vi "StateTurret.vi"(0 "Master State":enum16{"Normal", "Climb"}(ring)) -> ()   [LabVIEW 2020]
doc: "Performs all of the caluclations and decisions related to the turret."
uses:
  sensordata.vi
  robotoutputs.vi
panel:
  in  "Soft Limit A":dbl=125.0
  in  "Soft Limit B":dbl=-139.0
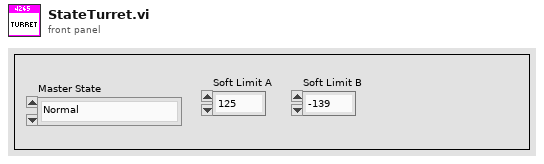
[diagram p1: front panel]
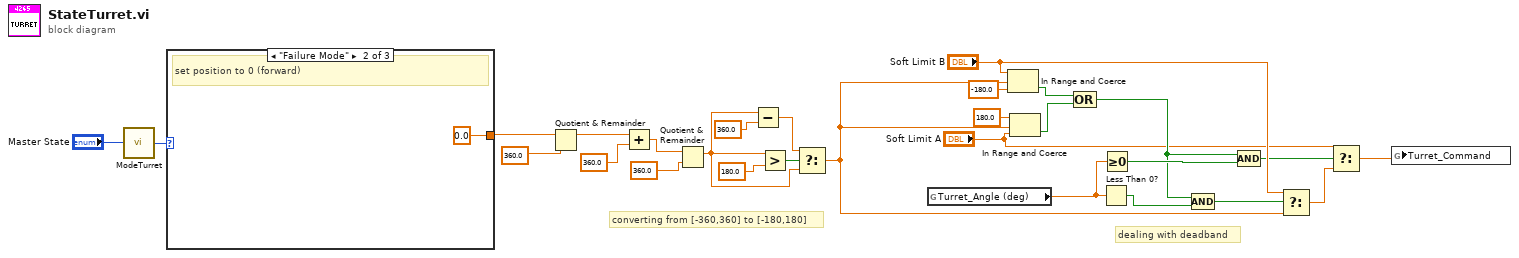
[diagram p0: block diagram]
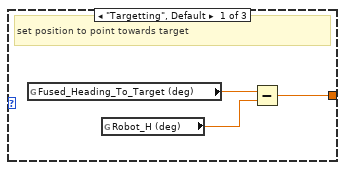
[diagram p2: hidden frame]
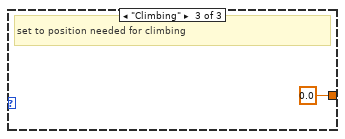
[diagram p3: hidden frame]
diagram:
  # "dealing with deadband"
  # "converting from [-360,360] to [-180,180]"
  n1 = call "ModeTurret.vi"("Master State"="Master State") -> ("Turret Mode"=w28:enum16{"Targetting", "Failure Mode", "Climbing"})
  n2 = case shown="\"Failure Mode\"" w28 {
    tunnel: [w30 0.0 0.0] -> w6
    frame "Targetting", Default {
      # "set position to point towards target"
      n3 = global read "sensordata.vi" "Fused_Heading_To_Target (deg)"() -> (w29:dbl)
      n4 = global read "sensordata.vi" "Robot_H (deg)"() -> (w31:dbl)
      n5 = Subtract(x=w29, y=w31) -> (x-y=w30:dbl)
    }
    frame "Failure Mode" {
      # "set position to 0 (forward)"
    }
    frame "Climbing" {
      # "set to position needed for climbing"
    }
  }
  n6 = Quotient & Remainder(x=w6, y=360.0) -> (x-y*floor(x/y)=w16:dbl)  [unwired: 1 out]
  n7 = Add(x=w16, y=360.0) -> (x+y=w14:dbl)
  n8 = Quotient & Remainder(x=w14, y=360.0) -> (x-y*floor(x/y)=w8:dbl)  [unwired: 1 out]
  n9 = Subtract(x=w8, y=360.0) -> (x-y=w9:dbl)
  n10 = Greater?(x=w8, y=180.0) -> (0:w11:bool)
  n11 = Select(t=w9, s=w11, f=w8) -> (s? t:f=w3:dbl)
  n12 = global read "sensordata.vi" "Turret_Angle (deg)"() -> (w7:dbl)
  n13 = In Range and Coerce(upper limit="Soft Limit B", x=w3, lower limit=-180.0) -> (In Range?=w24:bool)  [unwired: 1 out]
  n14 = In Range and Coerce(upper limit=180.0 ("lower limit"), x=w3, lower limit="Soft Limit A") -> (In Range?=w23:bool)  [unwired: 1 out]
  n15 = Compound Arithmetic op=OR(w24, w23) -> (w22:bool)
  n16 = Less Than 0?(x=w7) -> (x < 0?=w21:bool)
  n17 = Greater Or Equal To 0?(x=w7) -> (x >= 0?=w27:bool)
  n18 = Compound Arithmetic op=AND(w22, w21) -> (w4:bool)
  n19 = Compound Arithmetic op=AND(w22, w27) -> (w18:bool)
  n20 = Select(t="Soft Limit B", s=w4, f=w3) -> (s? t:f=w19:dbl)
  n21 = Select(t="Soft Limit A", s=w18, f=w19) -> (s? t:f=w2:dbl)
  n22 = global write "robotoutputs.vi" "Turret_Command"(w2) -> ()
